vi "DemultiplexV2.vi"(8 "Error In":errorcluster, 9 "General HardWare Constants":T1={"Nr. of Columns"=0, "Nr. of Rows"=0, "OverSampling"=0, "Fetch Rate "=0, "Sampling Rate"=0, "Nr. of BNC inputs"=3, "Sample Strip Length"=10}, 10 "Lookup Table":i32[](array[numeric]), 11 "Data In":dbl[][](array[numeric])=[[1.0, 3.0, 5.0, 7.0, 2.0], [1.0, 3.0, 5.0, 7.0, 2.0], [2.0, 4.0, 6.0, 8.0, 5.0], [2.0, 4.0, 6.0, 8.0, 5.0], [11.0, 33.0, 55.0, 77.0, 9.0], [11.0, 33.0, 55.0, 77.0, 9.0], [22.0, 44.0, 66.0, 88.0, 10.0], [22.0, 44.0, 66.0, 88.0, 10.0], [66.0, 77.0, 111.0, 333.0, 555.0], [66.0, 77.0, 111.0, 333.0, 555.0], [99.0, 88.0, 222.0, 444.0, 666.0], [99.0, 88.0, 222.0, 444.0, 666.0]]) -> (0 "Error Out":errorcluster, 1 "Data Out":dbl[][](array[numeric]))   [LabVIEW 2012]
uses:
  controls/General Hardware config.ctl
  <vilib>/Analysis/baseanly.llb/Mean (DBL).vi
  <vilib>/Analysis/NI_AALBase.lvlib
panel:
  # "Array"
  # "Acq. System"
  # "Other analog Input"
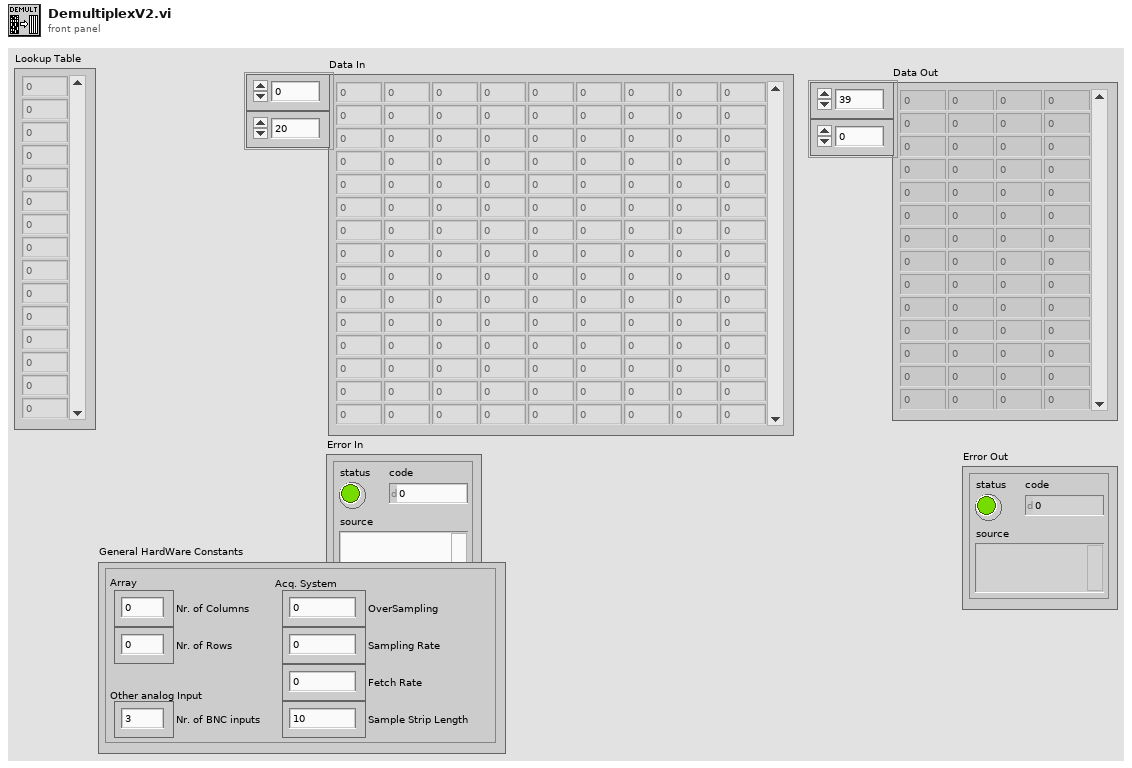
[diagram p1: front panel]
types:
  T1 = typedef "General Hardware config.ctl" = cluster{"Nr. of Columns":i32, "Nr. of Rows":i32, "OverSampling":i32, "Fetch Rate ":i32, "Sampling Rate":i32, "Nr. of BNC inputs":i32, "Sample Strip Length":i32}
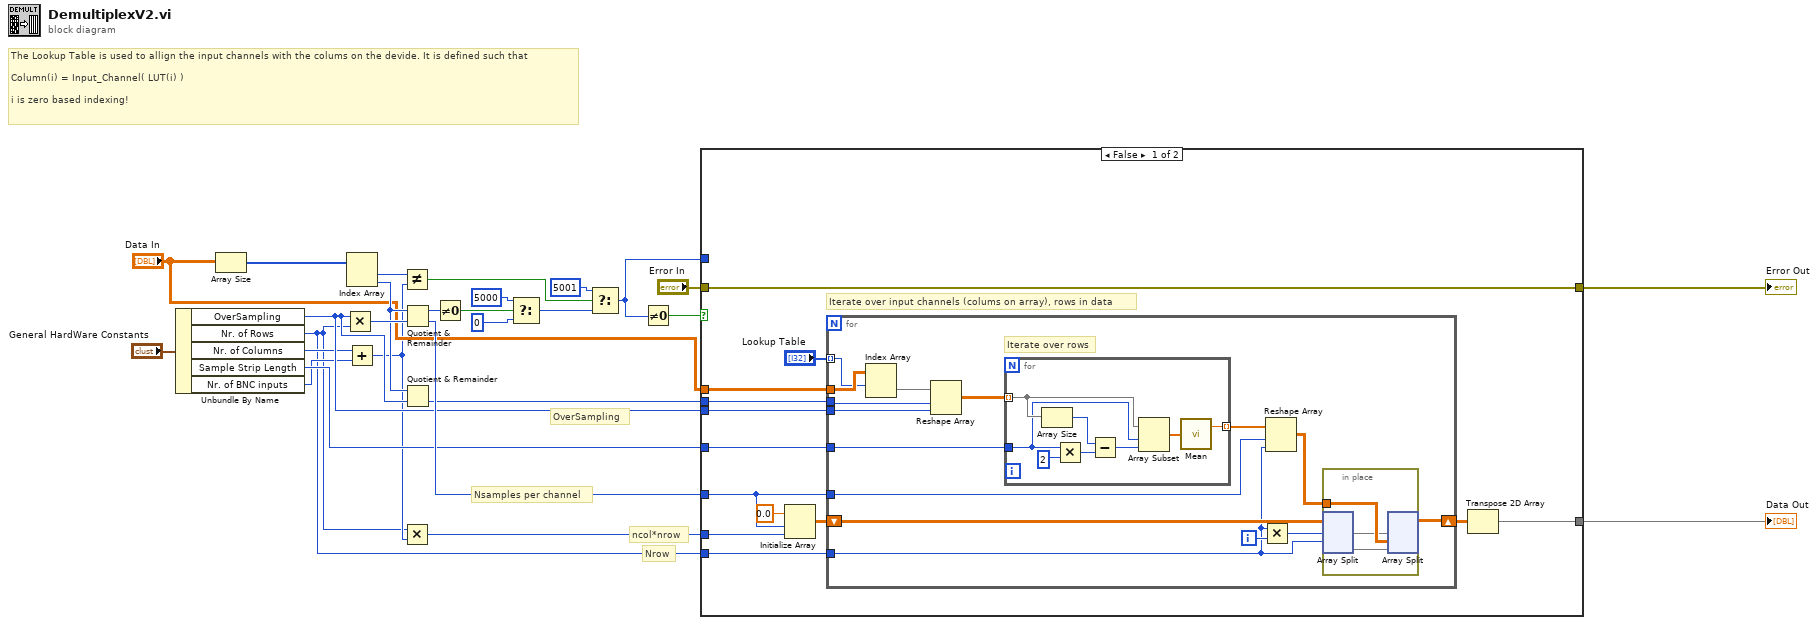
[diagram p0: block diagram]
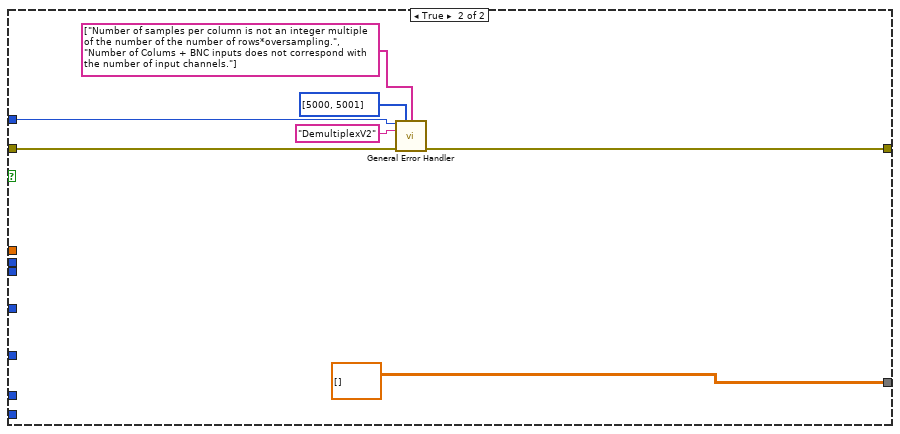
[diagram p2: hidden frame]
diagram:
  # "The Lookup Table is used to allign the input channels with the colums on the devide. It is defined such that \n\nColumn(i) = Input_Channel( LUT(i) )\n\ni is zero based indexing!"
  # "OverSampling"
  # "Nsamples per channel"
  # "Nrow"
  # "ncol*nrow"
  n1 = Unbundle By Name("General HardWare Constants") -> ("OverSampling"=w9:i32, "Nr. of Rows"=w2:i32, "Nr. of Columns"=w4:i32, "Sample Strip Length"=w6:i32, "Nr. of BNC inputs"=w5:i32)
  n2 = Array Size(array="Data In") -> (size(s)=w26:i32[])
  n3 = Multiply(x=w9, y=w2) -> (x*y=w16:i32)
  n4 = Index Array(array=w26) -> (element #1=w13:i32, element #2=w10:i32)  [unwired: 2 in]
  n5 = Add(x=w4, y=w5) -> (x+y=w3:i32)
  n6 = Not Equal?(x=w13, y=w3) -> (x != y?=w23:bool)
  n7 = Multiply(x=w2, y=w3) -> (x*y=w27:i32)
  n8 = Quotient & Remainder(x=w10, y=w16) -> (x-y*floor(x/y)=w14:i32, floor(x/y)=w11:i32)
  n9 = Quotient & Remainder(x=w10, y=w9) -> (floor(x/y)=w8:i32)  [unwired: 1 out]
  n10 = Not Equal To 0?(x=w14) -> (x != 0?=w15:bool)
  n11 = Select(t=i16 5000, s=w15, f=i16 0) -> (s? t:f=w17:i16)
  n12 = Select(t=i16 5001, s=w23, f=w17) -> (s? t:f=w12:i16)
  n13 = Not Equal To 0?(x=w12) -> (x != 0?=w21:bool)
  n14 = case shown="False" w21 {
    tunnel: w27 -> [w31 _]
    tunnel: "Data In" -> [w29 _]
    tunnel: [w30 dbl[][] []] -> w1
    tunnel: "Error In" -> [w37 w69]
    tunnel: [w37 w68] -> w25
    tunnel: w6 -> [w36 _]
    tunnel: w12 -> [_ w67]
    tunnel: w11 -> [w32 _]
    tunnel: w9 -> [w35 _]
    tunnel: w2 -> [w34 _]
    tunnel: w8 -> [w33 _]
    frame False {
      # "Iterate over input channels (colums on array), rows in data"
      n15 = Initialize Array(0.0 ("element"), w32, w31) -> (w39:dbl[][])
      n16 = for {
        shift-right: [w54] -> w38
        shift-left: w39 -> [w55]
        tunnel: w29 -> [w43]
        tunnel: w36 -> [w52]
        tunnel: w35 -> [w47]
        tunnel: w32 -> [w49]
        tunnel: w34 -> [w48]
        tunnel: w33 -> [w46]
        tunnel: "Lookup Table" -> [w42] mode=indexing
        i -> [w51]
        # "Iterate over rows"
        n17 = Index Array(array=w43, index (row)=w42) -> (element=w41:dbl[])  [unwired: 1 in]
        n18 = Reshape Array(w41, w46, w47) -> (w45:dbl[][])
        n19 = for {
          tunnel: w45 -> [w64] mode=indexing
          tunnel: [w66] -> w50 mode=indexing
          tunnel: w52 -> [w60]
          n20 = Array Size(array=w64) -> (size(s)=w63:i32)
          n21 = Multiply(x=w60, y=2) -> (x*y=w59:i32)
          n22 = Subtract(x=w63, y=w59) -> (x-y=w62:i32)
          n23 = Array Subset(array=w64, index=w60, length=w62) -> (w65:dbl[])
          n24 = call-poly <vilib>:"Mean.vi"("X"=w65) -> ("mean"=w66:dbl)  [unwired: 1 out]
        }
        n25 = Multiply(x=w48, y=w51) -> (x*y=w53:i32)
        n26 = Reshape Array(w50, w49, w48) -> (w44:dbl[][])
        n27 = in-place {
          in-place-border: w44 -> [w58]
          n28 = in-place-split #1(w55, w53, w48) -> (w56:dbl[][], w57:dbl[][])  [unwired: 1 out]
          n29 = in-place-split #1(w56, w58, w57) -> (w54:dbl[][])  [unwired: 2 out]
        }
      }
      n30 = Transpose 2D Array(2D array=w38) -> (transposed array=w30:dbl[][])
    }
    frame True {
      n31 = call <vilib>:"General Error Handler.vi"("[error code] (0)"=w67, "[user-defined codes]"=i32[] [5000, 5001], "[user-defined descriptions]"=string[] ["Number of samples per column is not an integer multiple of the number of the number of rows*oversampling.", "Number of Colums + BNC inputs does not correspond with the number of input channels."], "[error source] (\" \")"="DemultiplexV2" ("[error source] (\" \")"), "error in (no error)"=w69) -> ("error out"=w68:errorcluster)  [unwired: 6 in, 4 out]
    }
  }
  "Data Out" <- w1
  "Error Out" <- w25
